vi "WFS Configure Cam.vi"(8 "error in (no error)":errorcluster {"code" format="%.0x"}, 9 "Cam Resol. Index (1280x1024     640x480       1440x1080         1936x1216          2048x2048)":i32(ring) items=["1280x1024     640x480       1440x1080         1936x1216          2048x2048", "1024x1024     480x480       1080x1080         1216x1216          1536x1536", "768x768         360x360       768x768             1024x1024          1024x1024", "512x512         260x260       512x512             768x768              768x768    ", "320x320         180x180       360x360             512x512              512x512    ", "bin2 720x540         360x360              360x360    ", "bin2 540x540    sub2 968x608  sub2 1024x1024", "bin2 384x384    sub2 608x608      sub2 768x768", "bin2 256x256    sub2 512x512      sub2 512x512", "bin2 180x180    sub2 384x384      sub2 384x384", "sub2 256x256      sub2 256x256", "sub2 180x180      sub2 180x180"], 10 "Pixel Format (8 bit)":i32(ring) items=["16 bit"=1, "8 bit"=0], 11 "instrument handle":refnum<visa-resource-name>) -> (0 "error out":errorcluster {"code" format="%.0x"}, 1 "Spots Y":i32, 2 "Spots X":i32, 3 "instrument handle out":refnum<visa-resource-name>)   [LabVIEW 2020]
doc: "This VI configures the WFS instrument's camera resolution and returns the max. number of detectable spots in X and Y direction.\n\nThe result depends on the selected microlens array in WFS Select Mla.vi().\n\nNote: This VI is not available in Highspeed Mode!"
uses:
  WFS_32.dll
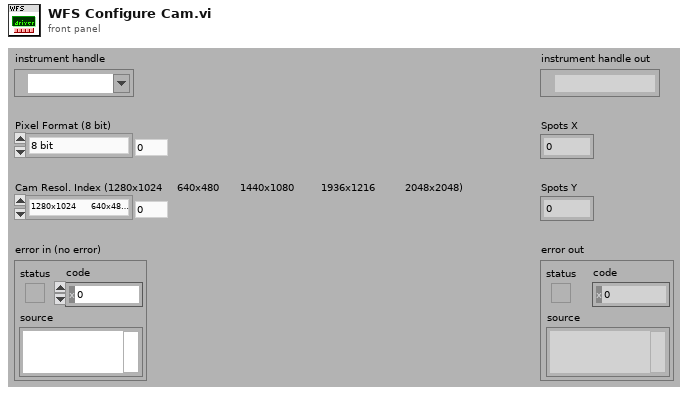
[diagram p1: front panel]
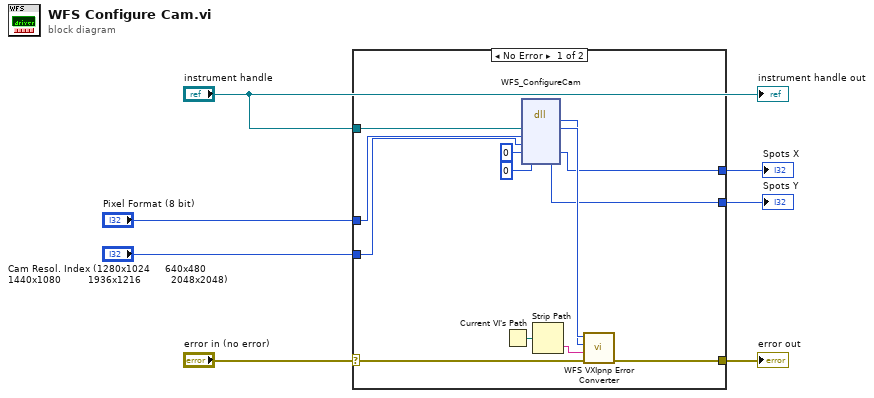
[diagram p0: block diagram]
diagram:
  n1 = case shown="No Error" "error in (no error)" {
    selector: "error in (no error)" -> [w15 w21]
    tunnel: [w14 w21] -> w7
    tunnel: "instrument handle" -> [w19 _]
    tunnel: "Pixel Format (8 bit)" -> [w13 _]
    tunnel: "Cam Resol. Index (1280x1024     640x480       1440x1080         1936x1216          2048x2048)" -> [w12 _]
    tunnel: [w10 _] -> w2
    tunnel: [w8 _] -> w1
    frame No Error {
      n2 = Current VI's Path() -> (path=w20:path)
      n3 = dll-call lib="WFS_*.*" fn="WFS_ConfigureCam"("Instrument Handle"=w19, "Pixel Format"=w13, "Cam Resol. Index"=w12, "Spots X"=0, "Spots Y"=0) -> (w17:i32, "Instrument Handle"=w18:u32, "Spots X"=w10:i32, "Spots Y"=w8:i32)  [unwired: 5 in, 2 out]
      n4 = Strip Path(path=w20) -> (name=w16:string)  [unwired: 1 out]
      n5 = call "WFS VXIpnp Error Converter.vi"("error in (no error)"=w15, "Name Of VI (\"\")"=w16, "CVI Error Code (0)"=w17, "instrument handle"=w18) -> ("error out"=w14:errorcluster)  [unwired: 6 in, 1 out]
    }
    frame Error {
    }
  }
  "error out" <- w7
  "Spots X" <- w2
  "Spots Y" <- w1
  "instrument handle out" <- "instrument handle"
